vi "Legacy IO Send Batch Commands.vi"(8 "error in":errorcluster, 11 "Legacy Commands Array":cluster{string, variant[]}[](array[cluster])) -> (0 "error out":errorcluster)   [LabVIEW 2011]
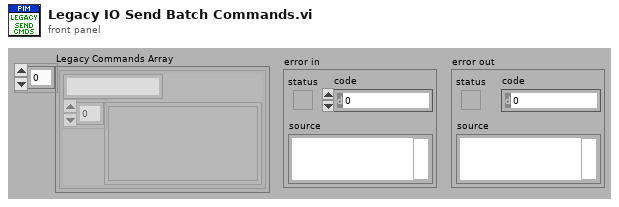
[diagram p1: front panel]
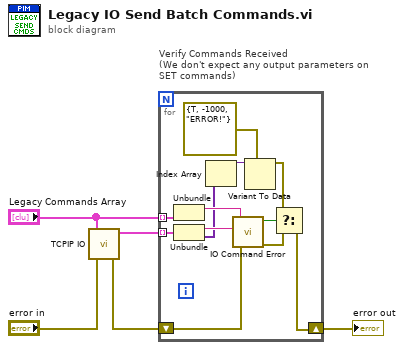
[diagram p0: block diagram]
diagram:
  n1 = call "TCPIP IO.vi"("error in (no error)"="error in", "Commands"="Legacy Commands Array") -> ("error out"=w4:errorcluster, "Responses"=w2:cluster{string, variant[]}[])  [unwired: 1 in, 3 out]
  n2 = for "Verify Commands Received\n(We don't expect any output parameters on SET commands)" {
    tunnel: w2 -> [w16] mode=indexing
    tunnel: "Legacy Commands Array" -> [w17] mode=indexing
    shift-right: [w7] -> w5
    shift-left: w4 -> [w13]
    n3 = Unbundle(w17) -> (w15:string)  [unwired: 1 out]
    n4 = Unbundle(w16) -> (w14:string, w6:variant[])
    n5 = Index Array(array=w6) -> (element=w11:variant)  [unwired: 1 in]
    n6 = call "IO Command Error.vi"("error in (no error)"=w13, "Command Returned (\"\")"=w14, "Command Sent (\"\")"=w15) -> ("error out"=w8:errorcluster, "HW ERR?"=w10:bool)  [unwired: 3 out]
    n7 = Variant To Data(type=errorcluster {"status"=TRUE, "code"=-1000, "source"="ERROR!"} ("error out"), Variant=w11) -> (data=w9:errorcluster)  [unwired: 1 in, 1 out]
    n8 = Select(t=w9, s=w10, f=w8) -> (s? t:f=w7:errorcluster)
  }
  "error out" <- w5
